vi "Input parameter to hex.vi"(7 "Function_In":string(combo)="Voltage", 9 "Value":dbl=264.0, 11 "Address(0x01)":u8 format="%.0x") -> (3 "Command(hex)":string)   [LabVIEW 2015]
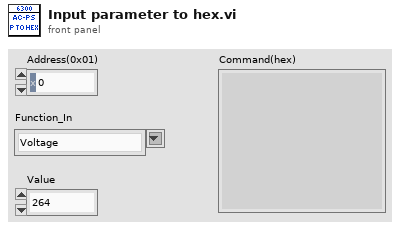
[diagram p1: front panel]
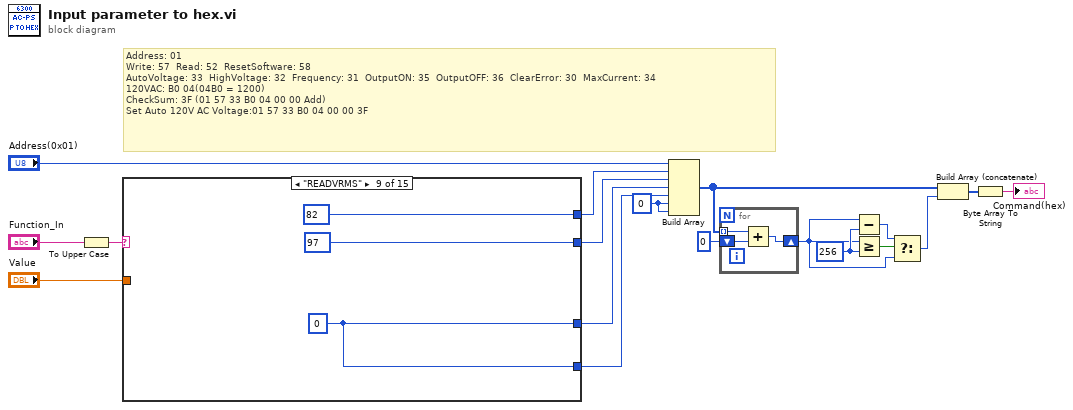
[diagram p0: block diagram]
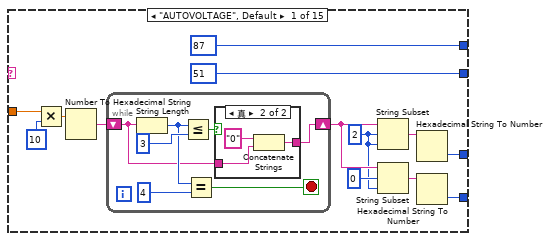
[diagram p2: hidden frame]
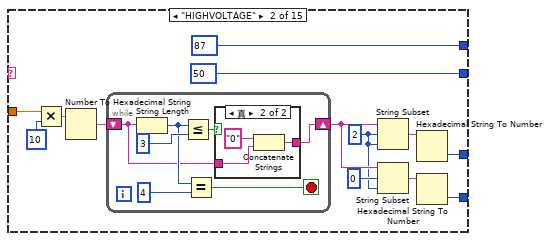
[diagram p4: hidden frame]
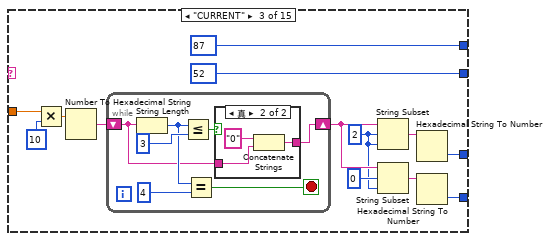
[diagram p6: hidden frame]
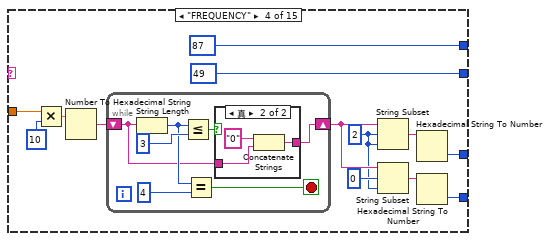
[diagram p8: hidden frame]
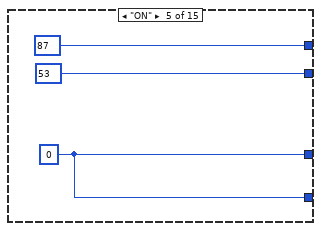
[diagram p10: hidden frame]
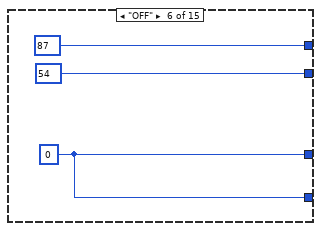
[diagram p11: hidden frame]
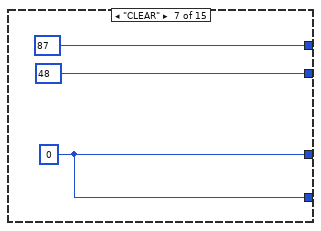
[diagram p12: hidden frame]
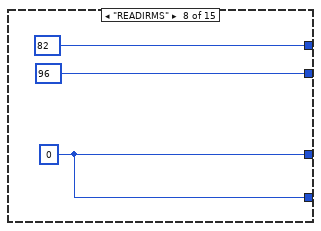
[diagram p13: hidden frame]
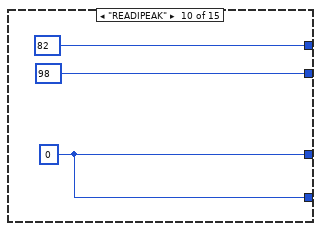
[diagram p14: hidden frame]
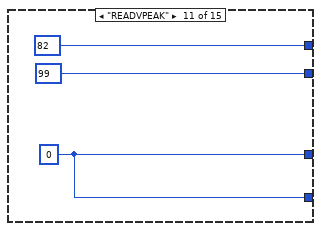
[diagram p15: hidden frame]
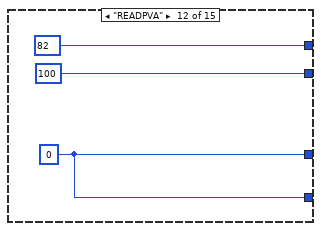
[diagram p16: hidden frame]
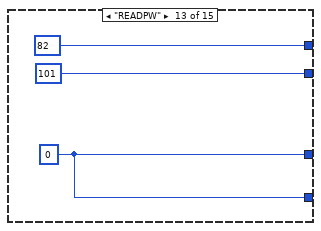
[diagram p17: hidden frame]
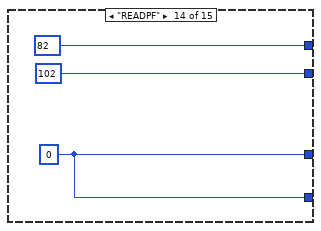
[diagram p18: hidden frame]
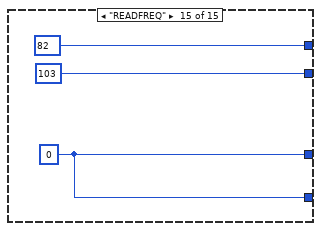
[diagram p19: hidden frame]
diagram:
  w6 = u32 256 ("y")
  w11 = u32 0 ("element")
  # "Address: 01\nWrite: 57  Read: 52  ResetSoftware: 58\nAutoVoltage: 33  HighVoltage: 32  Frequency: 31  OutputON: 35  OutputOFF: 36  ClearError: 30  MaxCurrent: 34\n120VAC: B0 04(04B0 = 1200)\nCheckSum: 3F (01 57 33 B0 04 00 00 Add)\nSet Auto 120V AC Voltage:01 57 33 B0 04 00 00 3F"
  n1 = To Upper Case(1:"Function_In") -> (0:w16:string)
  n2 = case shown="\"READVRMS\"" w16 {
    tunnel: [u8 51 ("element") u8 50 ("element") u8 52 ("element") u8 49 ("element") u8 53 ("element") u8 54 ("element") u8 48 ("element") u8 96 ("element") u8 97 ("element") u8 98 ("element") u8 99 ("element") u8 100 ("element") u8 101 ("element") u8 102 ("element") u8 103 ("element")] -> w15
    tunnel: "Value" -> [w24 w48 w72 w96 _ _ _ _ _ _ _ _ _ _ _]
    tunnel: [w23 w47 w71 w95 w115 w118 w121 w124 w127 w130 w133 w136 w139 w142 w145] -> w13
    tunnel: [w22 w46 w70 w94 w115 w118 w121 w124 w127 w130 w133 w136 w139 w142 w145] -> w12
    tunnel: [u8 87 ("element") u8 87 ("element") u8 87 ("element") u8 87 ("element") u8 87 ("element") u8 87 ("element") u8 87 ("element") u8 82 ("element") u8 82 ("element") u8 82 ("element") u8 82 ("element") u8 82 ("element") u8 82 ("element") u8 82 ("element") u8 82 ("element")] -> w10
    frame "AUTOVOLTAGE", Default {
      w20 = 2 ("offset (0)")
      n3 = Multiply(x=w24, y=u16 10) -> (x*y=w26:dbl)
      n4 = Number To Hexadecimal String(2:w26) -> (0:w27:string)  [unwired: 1 in]
      n5 = while {
        shift-right: [w32] -> w30
        shift-left: w27 -> [w33]
        stop <- w34 stop-if-true
        n6 = String Length(string=w33) -> (length=w36:i32)
        n7 = Less Or Equal?(x=w36, y=3) -> (x <= y?=w37:bool)
        n8 = Equal?(x=w36, y=4) -> (x = y?=w34:bool)
        n9 = case shown="真" w37 {
          tunnel: w33 -> [w39 w41]
          tunnel: [w39 w40] -> w32
          frame False {
          }
          frame True {
            n10 = Concatenate Strings("0", w41) -> (w40:string)
          }
        }
      }
      n11 = String Subset(string=w30, offset (0)=w20, length (rest)=w20) -> (substring=w28:string)
      n12 = String Subset(string=w30, offset (0)=0, length (rest)=w20) -> (substring=w29:string)
      n13 = Hexadecimal String To Number(string=w28) -> (number=w23:u32)  [unwired: 2 in, 1 out]
      n14 = Hexadecimal String To Number(string=w29) -> (number=w22:u32)  [unwired: 2 in, 1 out]
    }
    frame "HIGHVOLTAGE" {
      w44 = 2 ("offset (0)")
      n15 = Multiply(x=w48, y=u16 10) -> (x*y=w50:dbl)
      n16 = Number To Hexadecimal String(2:w50) -> (0:w51:string)  [unwired: 1 in]
      n17 = while {
        shift-right: [w56] -> w54
        shift-left: w51 -> [w57]
        stop <- w58 stop-if-true
        n18 = String Length(string=w57) -> (length=w60:i32)
        n19 = Less Or Equal?(x=w60, y=3) -> (x <= y?=w61:bool)
        n20 = Equal?(x=w60, y=4) -> (x = y?=w58:bool)
        n21 = case shown="真" w61 {
          tunnel: w57 -> [w63 w65]
          tunnel: [w63 w64] -> w56
          frame False {
          }
          frame True {
            n22 = Concatenate Strings("0", w65) -> (w64:string)
          }
        }
      }
      n23 = String Subset(string=w54, offset (0)=w44, length (rest)=w44) -> (substring=w52:string)
      n24 = String Subset(string=w54, offset (0)=0, length (rest)=w44) -> (substring=w53:string)
      n25 = Hexadecimal String To Number(string=w52) -> (number=w47:u32)  [unwired: 2 in, 1 out]
      n26 = Hexadecimal String To Number(string=w53) -> (number=w46:u32)  [unwired: 2 in, 1 out]
    }
    frame "CURRENT" {
      w68 = 2 ("offset (0)")
      n27 = Multiply(x=w72, y=u16 10) -> (x*y=w74:dbl)
      n28 = Number To Hexadecimal String(2:w74) -> (0:w75:string)  [unwired: 1 in]
      n29 = while {
        shift-right: [w80] -> w78
        shift-left: w75 -> [w81]
        stop <- w82 stop-if-true
        n30 = String Length(string=w81) -> (length=w84:i32)
        n31 = Less Or Equal?(x=w84, y=3) -> (x <= y?=w85:bool)
        n32 = Equal?(x=w84, y=4) -> (x = y?=w82:bool)
        n33 = case shown="真" w85 {
          tunnel: w81 -> [w87 w89]
          tunnel: [w87 w88] -> w80
          frame False {
          }
          frame True {
            n34 = Concatenate Strings("0", w89) -> (w88:string)
          }
        }
      }
      n35 = String Subset(string=w78, offset (0)=w68, length (rest)=w68) -> (substring=w76:string)
      n36 = String Subset(string=w78, offset (0)=0, length (rest)=w68) -> (substring=w77:string)
      n37 = Hexadecimal String To Number(string=w76) -> (number=w71:u32)  [unwired: 2 in, 1 out]
      n38 = Hexadecimal String To Number(string=w77) -> (number=w70:u32)  [unwired: 2 in, 1 out]
    }
    frame "FREQUENCY" {
      w92 = 2 ("offset (0)")
      n39 = Multiply(x=w96, y=u16 10) -> (x*y=w98:dbl)
      n40 = Number To Hexadecimal String(2:w98) -> (0:w99:string)  [unwired: 1 in]
      n41 = while {
        shift-right: [w104] -> w102
        shift-left: w99 -> [w105]
        stop <- w106 stop-if-true
        n42 = String Length(string=w105) -> (length=w108:i32)
        n43 = Less Or Equal?(x=w108, y=3) -> (x <= y?=w109:bool)
        n44 = Equal?(x=w108, y=4) -> (x = y?=w106:bool)
        n45 = case shown="真" w109 {
          tunnel: w105 -> [w111 w113]
          tunnel: [w111 w112] -> w104
          frame False {
          }
          frame True {
            n46 = Concatenate Strings("0", w113) -> (w112:string)
          }
        }
      }
      n47 = String Subset(string=w102, offset (0)=w92, length (rest)=w92) -> (substring=w100:string)
      n48 = String Subset(string=w102, offset (0)=0, length (rest)=w92) -> (substring=w101:string)
      n49 = Hexadecimal String To Number(string=w100) -> (number=w95:u32)  [unwired: 2 in, 1 out]
      n50 = Hexadecimal String To Number(string=w101) -> (number=w94:u32)  [unwired: 2 in, 1 out]
    }
    frame "ON" {
      w115 = u32 0
    }
    frame "OFF" {
      w118 = u32 0
    }
    frame "CLEAR" {
      w121 = u32 0
    }
    frame "READIRMS" {
      w124 = u32 0
    }
    frame "READVRMS" {
      w127 = u32 0
    }
    frame "READIPEAK" {
      w130 = u32 0
    }
    frame "READVPEAK" {
      w133 = u32 0
    }
    frame "READPVA" {
      w136 = u32 0
    }
    frame "READPW" {
      w139 = u32 0
    }
    frame "READPF" {
      w142 = u32 0
    }
    frame "READFREQ" {
      w145 = u32 0
    }
  }
  n51 = Build Array("Address(0x01)", w10, w15, w13, w12, w11, w11) -> (w4:u32[])
  n52 = for {
    tunnel: w4 -> [w150] mode=indexing
    shift-right: [w149] -> w5
    shift-left: u32 0 -> [w148]
    n53 = Add(x=w150, y=w148) -> (x+y=w149:u32)
  }
  n54 = Subtract(x=w5, y=w6) -> (x-y=w7:u32)
  n55 = Greater Or Equal?(x=w5, y=w6) -> (x >= y?=w8:bool)
  n56 = Select(t=w7, s=w8, f=w5) -> (s? t:f=w3:u32)
  n57 = Build Array (concatenate)(w4, w3) -> (w2:u32[])
  n58 = Byte Array To String(unsigned byte array=w2) -> (string=→"Command(hex)":string)
